vi "Calculate Points of Line with diagonal.vi"(8 "Yf":i32, 9 "Yi":i32, 10 "Xf":i32, 11 "Xi":i32) -> (2 "Y Points":i32[](array[numeric]), 3 "X Points":i32[](array[numeric]))   [LabVIEW 2019, in "Day 5.lvlib"]
uses:
  Day 5.lvlib
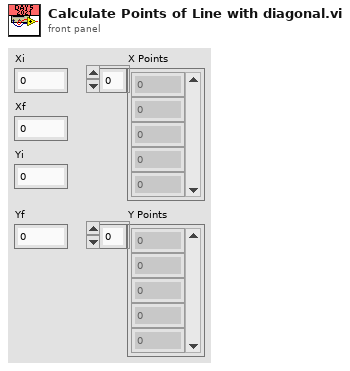
[diagram p1: front panel]
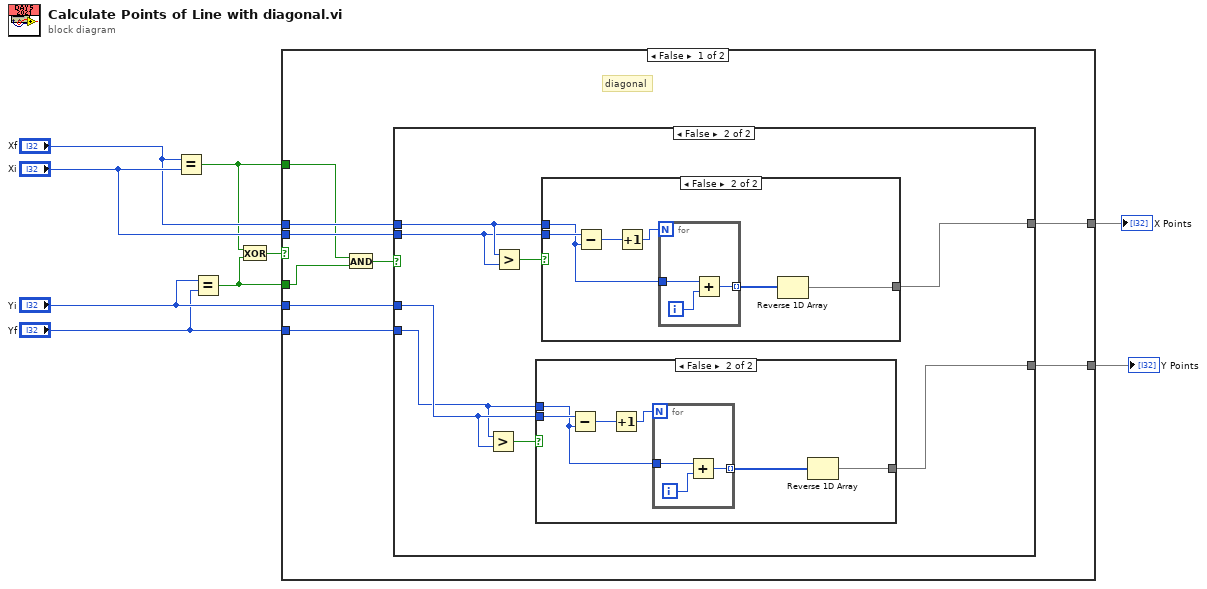
[diagram p0: block diagram]
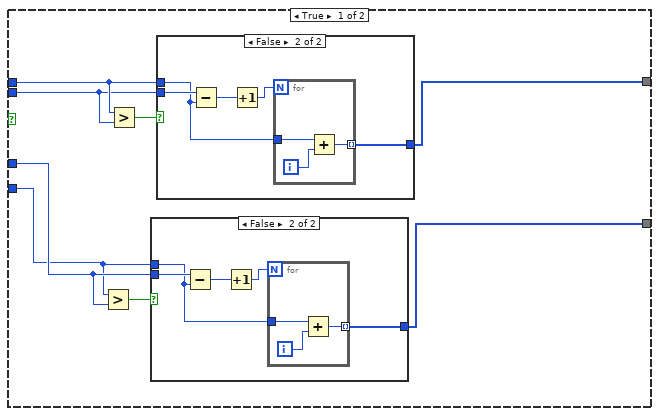
[diagram p2: hidden frame]
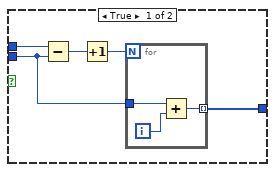
[diagram p3: hidden frame]
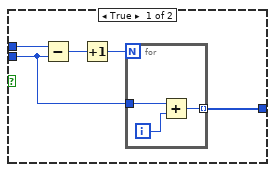
[diagram p4: hidden frame]
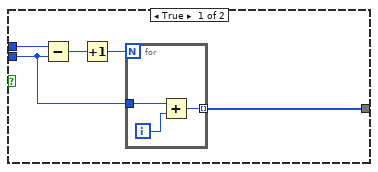
[diagram p5: hidden frame]
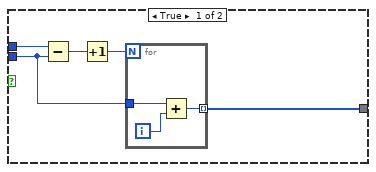
[diagram p6: hidden frame]
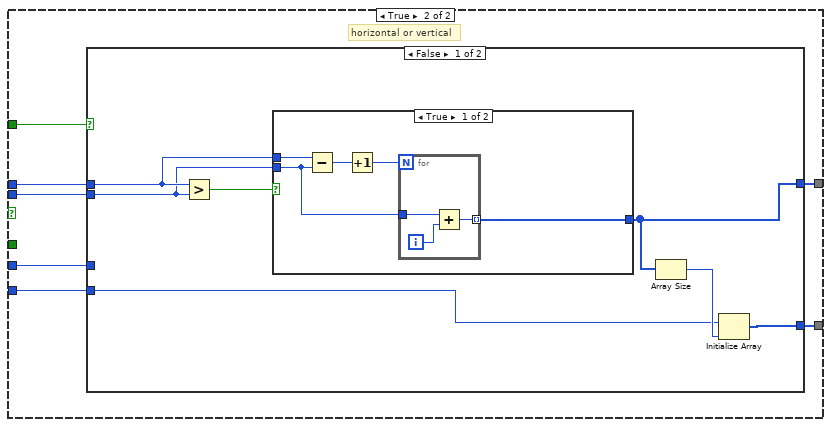
[diagram p7: hidden frame]
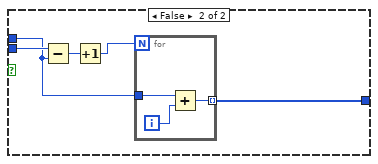
[diagram p8: hidden frame]
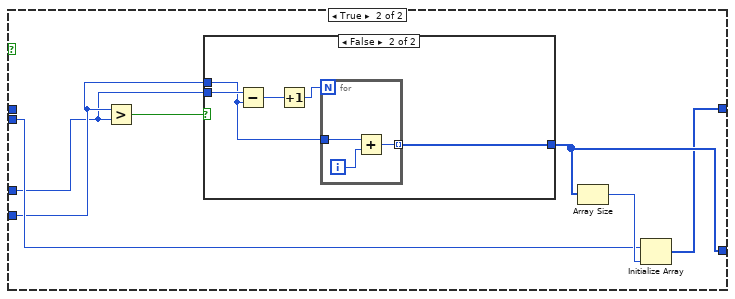
[diagram p9: hidden frame]
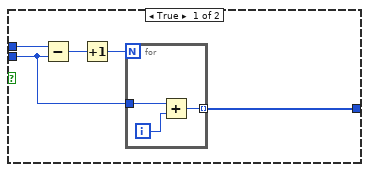
[diagram p10: hidden frame]
diagram:
  n1 = Equal?(x="Xf", y="Xi") -> (x = y?=w3:bool)
  n2 = Equal?(x="Yi", y="Yf") -> (x = y?=w1:bool)
  n3 = Exclusive Or(1:w1, 2:w3) -> (0:w2:bool)
  n4 = case shown="False" w2 {
    tunnel: w3 -> [w12 w107]
    tunnel: "Xi" -> [w14 w106]
    tunnel: "Xf" -> [w18 w105]
    tunnel: "Yi" -> [w17 w104]
    tunnel: "Yf" -> [w13 w103]
    tunnel: [w15 w102] -> w7
    tunnel: [w16 w101] -> w6
    tunnel: w1 -> [w11 _]
    frame False {
      # "diagonal"
      n5 = And(x=w12, y=w11) -> (x .and. y?=w10:bool)
      n6 = case shown="False" w10 {
        tunnel: w18 -> [w26 w66]
        tunnel: w17 -> [w25 w65]
        tunnel: [w24 w64] -> w16
        tunnel: [w23 w59] -> w15
        tunnel: w14 -> [w20 w61]
        tunnel: w13 -> [w19 w60]
        frame True {
          n7 = Greater?(x=w19, y=w25) -> (0:w21:bool)
          n8 = Greater?(x=w26, y=w20) -> (0:w22:bool)
          n9 = case shown="False" w21 {
            tunnel: w19 -> [w31 w37]
            tunnel: w25 -> [w30 w38]
            tunnel: [w29 w39] -> w23
            frame True {
              n10 = Subtract(x=w31, y=w30) -> (x-y=w28:i32)
              n11 = Increment(x=w28) -> (x+1=w27:i32)
              n12 = for {
                N: w27 -> [_]
                tunnel: w30 -> [w34]
                tunnel: [w32] -> w29 mode=indexing
                i -> [w33]
                n13 = Add(x=w34, y=w33) -> (x+y=w32:i32)
              }
            }
            frame False {
              n14 = Subtract(x=w38, y=w37) -> (x-y=w36:i32)
              n15 = Increment(x=w36) -> (x+1=w35:i32)
              n16 = for {
                N: w35 -> [_]
                tunnel: w37 -> [w42]
                tunnel: [w40] -> w39 mode=indexing
                i -> [w41]
                n17 = Add(x=w42, y=w41) -> (x+y=w40:i32)
              }
            }
          }
          n18 = case shown="False" w22 {
            tunnel: w26 -> [w47 w53]
            tunnel: w20 -> [w46 w54]
            tunnel: [w45 w55] -> w24
            frame True {
              n19 = Subtract(x=w47, y=w46) -> (x-y=w44:i32)
              n20 = Increment(x=w44) -> (x+1=w43:i32)
              n21 = for {
                N: w43 -> [_]
                tunnel: w46 -> [w50]
                tunnel: [w48] -> w45 mode=indexing
                i -> [w49]
                n22 = Add(x=w50, y=w49) -> (x+y=w48:i32)
              }
            }
            frame False {
              n23 = Subtract(x=w54, y=w53) -> (x-y=w52:i32)
              n24 = Increment(x=w52) -> (x+1=w51:i32)
              n25 = for {
                N: w51 -> [_]
                tunnel: w53 -> [w58]
                tunnel: [w56] -> w55 mode=indexing
                i -> [w57]
                n26 = Add(x=w58, y=w57) -> (x+y=w56:i32)
              }
            }
          }
        }
        frame False {
          n27 = Greater?(x=w60, y=w65) -> (0:w62:bool)
          n28 = Greater?(x=w66, y=w61) -> (0:w63:bool)
          n29 = case shown="False" w62 {
            tunnel: w60 -> [w71 w79]
            tunnel: w65 -> [w70 w80]
            tunnel: [w69 w75] -> w59
            frame True {
              n30 = Subtract(x=w71, y=w70) -> (x-y=w68:i32)
              n31 = Increment(x=w68) -> (x+1=w67:i32)
              n32 = for {
                N: w67 -> [_]
                tunnel: w70 -> [w74]
                tunnel: [w72] -> w69 mode=indexing
                i -> [w73]
                n33 = Add(x=w74, y=w73) -> (x+y=w72:i32)
              }
            }
            frame False {
              n34 = Subtract(x=w80, y=w79) -> (x-y=w78:i32)
              n35 = Increment(x=w78) -> (x+1=w77:i32)
              n36 = for {
                N: w77 -> [_]
                tunnel: w79 -> [w83]
                tunnel: [w81] -> w76 mode=indexing
                i -> [w82]
                n37 = Add(x=w83, y=w82) -> (x+y=w81:i32)
              }
              n38 = Reverse 1D Array(array=w76) -> (reversed array=w75:i32[])
            }
          }
          n39 = case shown="False" w63 {
            tunnel: w66 -> [w88 w96]
            tunnel: w61 -> [w87 w97]
            tunnel: [w86 w92] -> w64
            frame True {
              n40 = Subtract(x=w88, y=w87) -> (x-y=w85:i32)
              n41 = Increment(x=w85) -> (x+1=w84:i32)
              n42 = for {
                N: w84 -> [_]
                tunnel: w87 -> [w91]
                tunnel: [w89] -> w86 mode=indexing
                i -> [w90]
                n43 = Add(x=w91, y=w90) -> (x+y=w89:i32)
              }
            }
            frame False {
              n44 = Subtract(x=w97, y=w96) -> (x-y=w95:i32)
              n45 = Increment(x=w95) -> (x+1=w94:i32)
              n46 = for {
                N: w94 -> [_]
                tunnel: w96 -> [w100]
                tunnel: [w98] -> w93 mode=indexing
                i -> [w99]
                n47 = Add(x=w100, y=w99) -> (x+y=w98:i32)
              }
              n48 = Reverse 1D Array(array=w93) -> (reversed array=w92:i32[])
            }
          }
        }
      }
    }
    frame True {
      # "horizontal or vertical"
      n49 = case shown="False" w107 {
        tunnel: w106 -> [w112 w133]
        tunnel: w105 -> [w113 _]
        tunnel: w104 -> [_ w131]
        tunnel: w103 -> [w110 w132]
        tunnel: [w108 w136] -> w102
        tunnel: [w109 w134] -> w101
        frame False {
          n50 = Greater?(x=w113, y=w112) -> (0:w114:bool)
          n51 = case shown="True" w114 {
            tunnel: w113 -> [w119 w125]
            tunnel: w112 -> [w118 w126]
            tunnel: [w117 w127] -> w109
            frame True {
              n52 = Subtract(x=w119, y=w118) -> (x-y=w116:i32)
              n53 = Increment(x=w116) -> (x+1=w115:i32)
              n54 = for {
                N: w115 -> [_]
                tunnel: w118 -> [w122]
                tunnel: [w120] -> w117 mode=indexing
                i -> [w121]
                n55 = Add(x=w122, y=w121) -> (x+y=w120:i32)
              }
            }
            frame False {
              n56 = Subtract(x=w126, y=w125) -> (x-y=w124:i32)
              n57 = Increment(x=w124) -> (x+1=w123:i32)
              n58 = for {
                N: w123 -> [_]
                tunnel: w125 -> [w130]
                tunnel: [w128] -> w127 mode=indexing
                i -> [w129]
                n59 = Add(x=w130, y=w129) -> (x+y=w128:i32)
              }
            }
          }
          n60 = Array Size(array=w109) -> (size(s)=w111:i32)
          n61 = Initialize Array(w110, w111) -> (w108:i32[])
        }
        frame True {
          n62 = Greater?(x=w132, y=w131) -> (0:w137:bool)
          n63 = case shown="False" w137 {
            tunnel: w132 -> [w142 w148]
            tunnel: w131 -> [w141 w149]
            tunnel: [w140 w150] -> w136
            frame True {
              n64 = Subtract(x=w142, y=w141) -> (x-y=w139:i32)
              n65 = Increment(x=w139) -> (x+1=w138:i32)
              n66 = for {
                N: w138 -> [_]
                tunnel: w141 -> [w145]
                tunnel: [w143] -> w140 mode=indexing
                i -> [w144]
                n67 = Add(x=w145, y=w144) -> (x+y=w143:i32)
              }
            }
            frame False {
              n68 = Subtract(x=w149, y=w148) -> (x-y=w147:i32)
              n69 = Increment(x=w147) -> (x+1=w146:i32)
              n70 = for {
                N: w146 -> [_]
                tunnel: w148 -> [w153]
                tunnel: [w151] -> w150 mode=indexing
                i -> [w152]
                n71 = Add(x=w153, y=w152) -> (x+y=w151:i32)
              }
            }
          }
          n72 = Array Size(array=w136) -> (size(s)=w135:i32)
          n73 = Initialize Array(w133, w135) -> (w134:i32[])
        }
      }
    }
  }
  "Y Points" <- w7
  "X Points" <- w6
